vi "Initialize.vi"(8 "error in":errorcluster, 10 "Device":string) -> (0 "error out":errorcluster, 3 "Optical Power Meter out":refnum<class "Optical Power Meter.lvclass">)   [LabVIEW 2018, in "Optical Power Meter.lvlib" / "Optical Power Meter.lvclass"]
uses:
  Optical Power Meter.lvclass
  Optical Power Meter.lvclass/Optical Power Meter.ctl
  PPLs/Configuration/Configuration.lvlibp/Configuration.lvclass
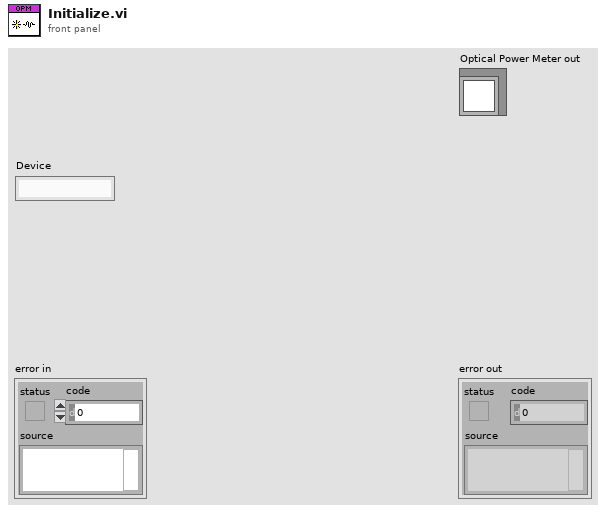
[diagram p1: front panel]
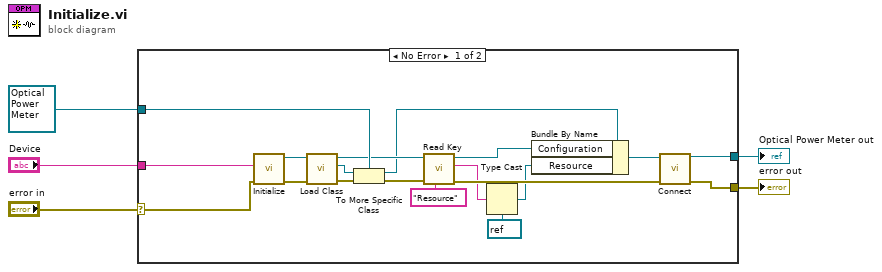
[diagram p0: block diagram]
diagram:
  n1 = case shown="No Error" "error in" {
    selector: "error in" -> [w10 w26]
    tunnel: [w9 w26] -> w4
    tunnel: [w12 w25] -> w2
    tunnel: refnum<class "Optical Power Meter.lvclass"> refnum ("Optical Power Meter in") -> [w19 w25]
    tunnel: "Device" -> [w24 _]
    frame No Error {
      n2 = call "Initialize.vi"("error in"=w10, "Device"=w24) -> ("error out"=w22:errorcluster, "Configuration out"=w23:refnum<class "Configuration.lvclass">)  [unwired: 8 in]
      n3 = call "Load Class.vi"("error in"=w22, "Configuration in"=w23) -> ("error out"=w21:errorcluster, "Class out"=w20:refnum<class>, "Configuration out"=w18:refnum<class "Configuration.lvclass">)  [unwired: 7 in]
      n4 = To More Specific Class(target class=w19, reference=w20, error in=w21) -> (specific class reference=w15:refnum<class "Optical Power Meter.lvclass">, error out=w16:errorcluster)
      n5 = call "Read Key.vi"("Key:"="Resource", "error in"=w16, "Configuration in"=w18) -> ("error out"=w11:errorcluster, "Value"=w7:string, "Configuration out"=w14:refnum<class "Configuration.lvclass">)  [unwired: 6 in]
      n6 = Type Cast(type=refnum<visa-resource-name> refnum ("Resource"), x=w7) -> (*(type *) &x=w6:refnum<visa-resource-name>)
      n7 = Bundle By Name(cluster=w15, "Configuration"=w14, "Resource"=w6) -> (w13:refnum<class "Optical Power Meter.lvclass">)
      n8 = call-dynamic "Connect.vi"("error in (no error)"=w11, "Optical Power Meter in"=w13) -> ("error out"=w9:errorcluster, "Optical Power Meter out"=w12:refnum<class "Optical Power Meter.lvclass">)  [unwired: 8 in]
    }
    frame Error {
    }
  }
  "error out" <- w4
  "Optical Power Meter out" <- w2
